vi "Password.vi"() -> ()   [LabVIEW 2019]
uses:
  lib/Snap7.lvlib
panel:
  out "?":string
  in  "stop":bool
  out "Result":i32
  in  "ClrPWD":bool
  in  "SetPWD":bool
  in  "Password":string
  out "Status":string
  in  "Slot":i32=2
  in  "Rack":i32
  in  "Address IP":string="192.168.1.12"
  # "Set Session Password"
  # "Clear Session Password"
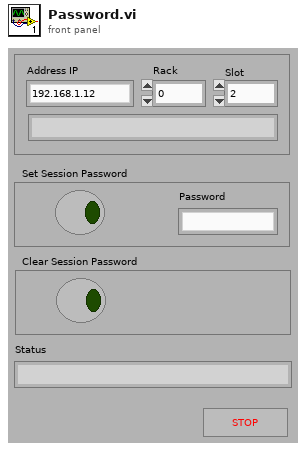
[diagram p1: front panel]
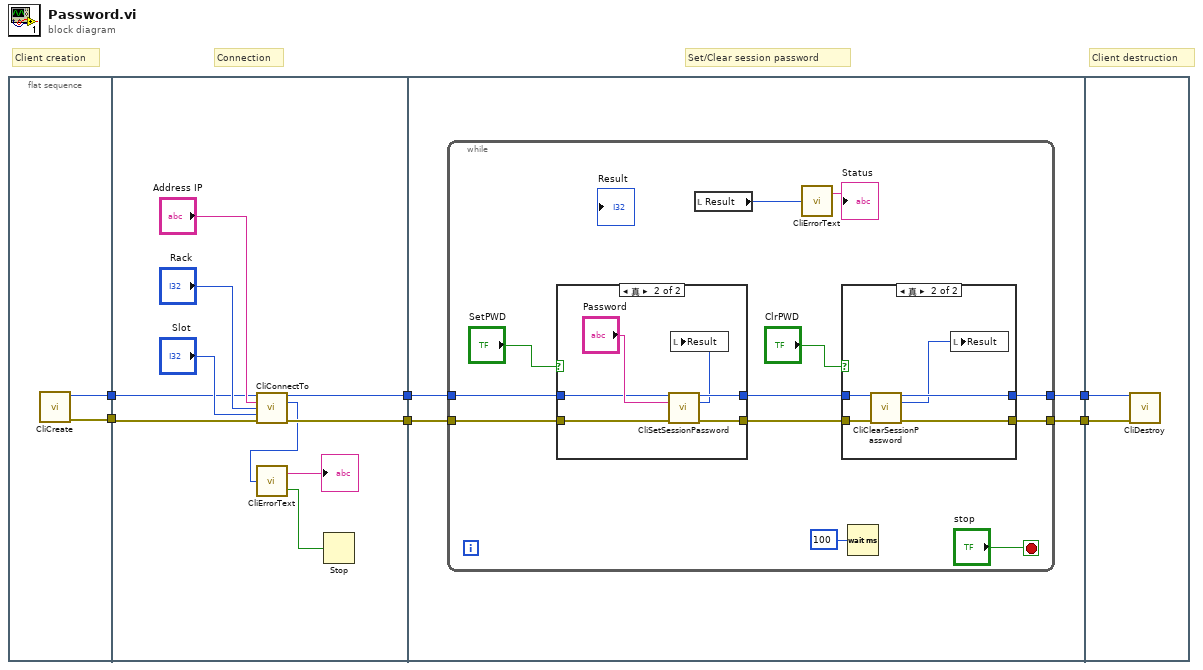
[diagram p0: block diagram]
diagram:
  # "Client destruction"
  # "Set/Clear session password"
  # "Connection"
  # "Client creation"
  n1 = flat-sequence {
    tunnel: [w8] -> w4
    tunnel: [w7] -> w3
    tunnel: [w18] -> w6
    tunnel: [w12] -> w5
    tunnel: w4 -> [w14]
    tunnel: w3 -> [w13]
    tunnel: w6 -> [w20]
    tunnel: w5 -> [w22]
    tunnel: [w21] -> w2
    tunnel: [w19] -> w1
    tunnel: w2 -> [w51]
    tunnel: w1 -> [w50]
    frame #0 {
      n2 = call "CliCreate.vi"() -> ("ref out"=w8:u64, "error out"=w7:errorcluster)  [unwired: 14 in]
    }
    frame #1 {
      n3 = call "CliConnectTo.vi"("ref in"=w14, "Address"="Address IP", "Rack"="Rack", "Slot"="Slot", "error in (no error)"=w13) -> ("ref out"=w12:u64, "Result"=w9:i32, "error out"=w18:errorcluster)  [unwired: 8 in]
      n4 = call "CliErrorText.vi"("ErrNo"=w9) -> ("Error"=w11:bool, "ErrMessage"=→"?":string)
      n5 = Stop(stop? (T)=w11) -> ()
    }
    frame #2 {
      n6 = while {
        tunnel: w22 -> [w34]
        tunnel: [w32] -> w21
        tunnel: w20 -> [w29]
        tunnel: [w27] -> w19
        stop <- "stop" stop-if-true
        n7 = case shown="真" "SetPWD" {
          tunnel: w34 -> [w43 w48]
          tunnel: [w43 w47] -> w33
          tunnel: w29 -> [w42 w46]
          tunnel: [w42 w45] -> w28
          frame False {
          }
          frame True {
            n8 = call "CliSetSessionPassword.vi"("ref in"=w48, "Password"="Password", "error in (no error)"=w46) -> ("ref out"=w47:u64, "Result"=w44:i32, "error out"=w45:errorcluster)  [unwired: 10 in]
            n9 = local write "Result"(w44) -> ()
          }
        }
        n10 = local read "Result"() -> (w25:i32)
        n11 = call "CliErrorText.vi"("ErrNo"=w25) -> ("ErrMessage"=→"Status":string)  [unwired: 1 out]
        n12 = case shown="真" "ClrPWD" {
          tunnel: w33 -> [w36 w41]
          tunnel: [w36 w40] -> w32
          tunnel: w28 -> [w35 w39]
          tunnel: [w35 w38] -> w27
          frame False {
          }
          frame True {
            n13 = call "CliClearSessionPassword.vi"("ref in"=w41, "error in (no error)"=w39) -> ("ref out"=w40:u64, "Result"=w37:i32, "error out"=w38:errorcluster)  [unwired: 11 in]
            n14 = local write "Result"(w37) -> ()
          }
        }
        n15 = Wait (ms)(milliseconds to wait=u32 100 ("Loop Delay (ms)")) -> ()  [unwired: 1 out]
      }
    }
    frame #3 {
      n16 = call "CliDestroy.vi"("ref in"=w51, "error in (no error)"=w50) -> ()  [unwired: 13 in, 1 out]
    }
  }
